vi "layout.vi"(0 "reference":refnum<class "CallNode.lvclass">, 1 "graph":refnum<class "Graph.lvclass">, 2 "graphics":refnum<class "Graphics.lvclass">, 3 "grid":refnum<class "Grid.lvclass">, 5 "error in (no error)":errorcluster) -> (14 "reference out":refnum<class "CallNode.lvclass">, 19 "error out":errorcluster)   [LabVIEW 2016, in "CallNode.lvclass"]
doc: "public void layout(Graph g, Graphics2D g2, Grid grid)"
uses:
  <resource>/Framework/Providers/Open_GDS/UML/CallNode_class/CallNode.lvclass
  C:/Program Files (x86)/National Instruments/LabVIEW 2016/resource/Framework/Providers/Open_GDS/UML/RectangularNode_class/RectangularNode.lvclass
  C:/Program Files (x86)/National Instruments/LabVIEW 2016/resource/Framework/Providers/Open_GDS/UML/AbstractNode_class/AbstractNode.lvclass
  <resource>/Framework/Providers/Open_GDS/UML/Graph_class/Graph.lvclass
  <resource>/Framework/Providers/Open_GDS/UML/Graphics_class/Graphics.lvclass
  <resource>/Framework/Providers/Open_GDS/UML/Grid_class/Grid.lvclass
  <resource>/Framework/Providers/Open_GDS/UML/ImplicitParameterNode_class/ImplicitParameterNode.lvclass
  <resource>/Framework/Providers/Open_GDS/UML/AbstractNode_class/AbstractNode.lvclass
  <resource>/Framework/Providers/Open_GDS/UML/RectangularNode_class/RectangularNode.lvclass
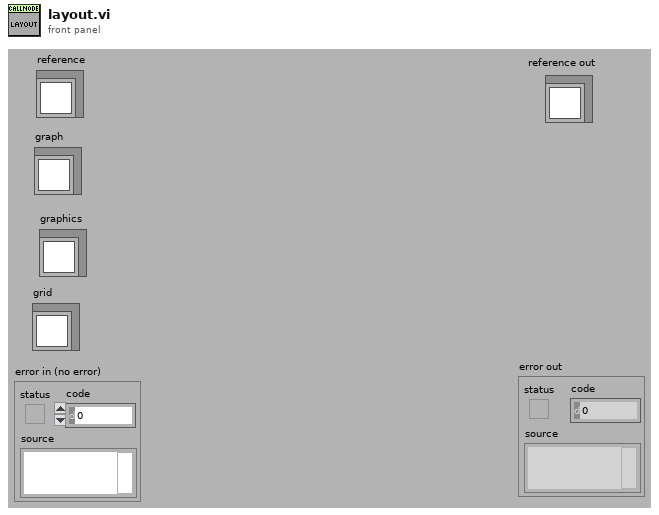
[diagram p1: front panel]
types:
  T1 = typedef "CallNode.lvclass/ObjectAttributes.ctl" = cluster{"objectCallNodeRef":refnum<class "AbstractNode.lvclass">, "signaled":bool, "openBottom":bool, "DEFAULT_WIDTH":i32, "DEFAULT_HEIGHT":i32, "CALL_YGAP":i32}
  T2 = typedef "RectangularNode.lvclass/ObjectAttributes.ctl" = cluster{"bounds":T3}
  T3 = typedef "Rectangle Rectangle2D.ctl" = cluster{"x":dbl, "y":dbl, "width":dbl, "height":dbl}
  T4 = typedef "AbstractNode.lvclass/ObjectAttributes.ctl" = cluster{"parent":refnum<class "AbstractNode.lvclass">, "children":refnum<class "AbstractNode.lvclass">[], "Hidden":bool}
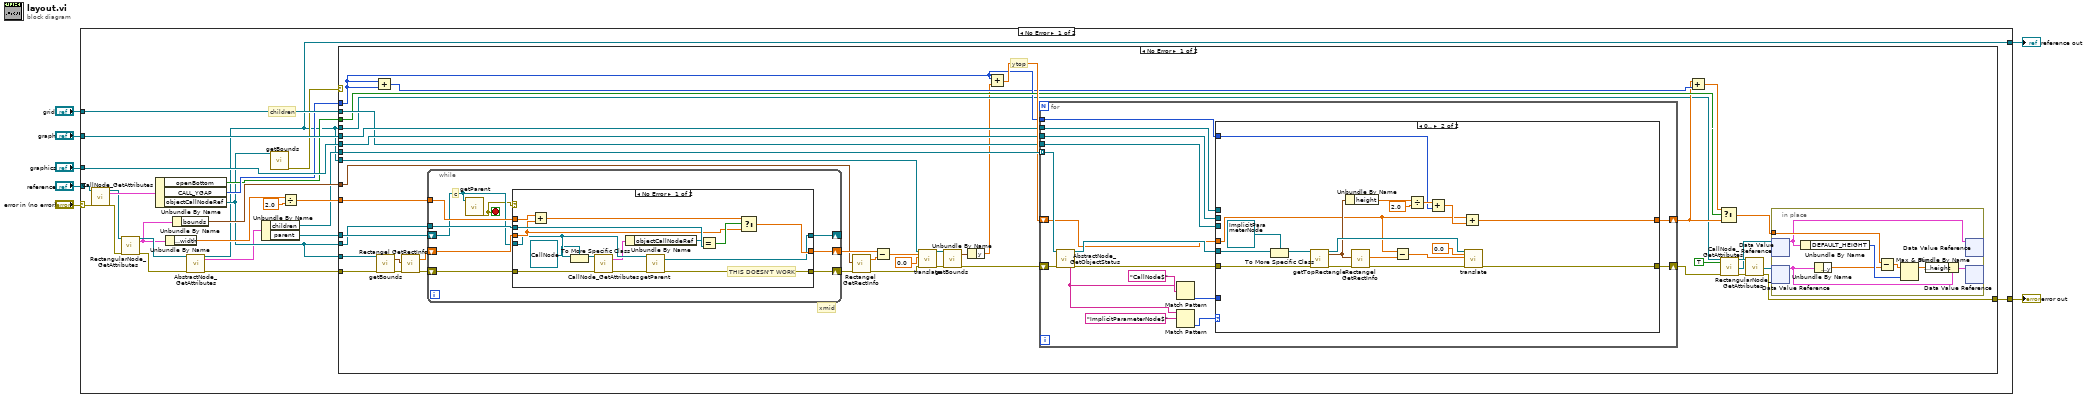
[diagram p0: block diagram]
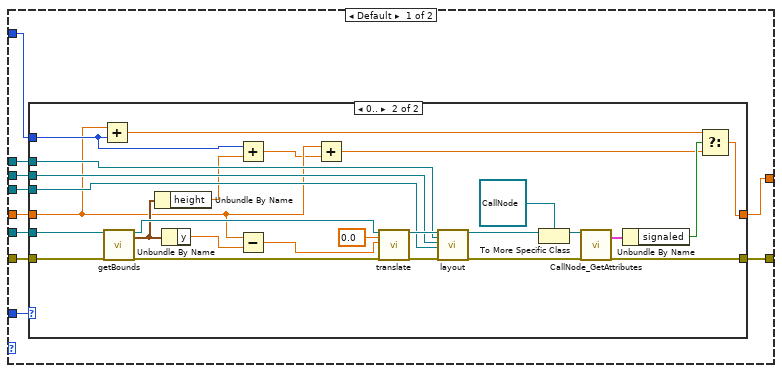
[diagram p2: hidden frame]
diagram:
  n1 = case shown="No Error" "error in (no error)" {
    selector: "error in (no error)" -> [w30 w184]
    tunnel: "reference" -> [w32 w185]
    tunnel: [w31 w184] -> w6
    tunnel: [w10 w185] -> w5
    tunnel: "graph" -> [w29 _]
    tunnel: "graphics" -> [w28 _]
    tunnel: "grid" -> [w27 _]
    frame No Error {
      # "children"
      n2 = call <resource>:"CallNode_GetAttributes.vi"("reference in"=w32, "error in (no error)"=w30) -> ("reference out"=w15:refnum<class "CallNode.lvclass">, "Data"=w16:T1, "error out"=w14:errorcluster)  [unwired: 1 in, 14 out]
      n3 = call <resource>:"RectangularNode_GetAttributes.vi"("reference in"=w15, "error in (no error)"=w14) -> ("reference out"=w13:refnum<class "CallNode.lvclass">, "Data"=w9:T2, "error out"=w12:errorcluster)  [unwired: 14 in, 1 out]
      n4 = Unbundle By Name(w16) -> ("openBottom"=w19:bool, "CALL_YGAP"=w21:i32, "objectCallNodeRef"=w17:refnum<class "AbstractNode.lvclass">)
      n5 = Unbundle By Name(w9) -> ("bounds.width"=w25:dbl)
      n6 = Unbundle By Name(w9) -> ("bounds"=w22:T3)
      n7 = call <resource>:"AbstractNode_GetAttributes.vi"("reference in"=w13, "error in (no error)"=w12) -> ("reference out"=w10:refnum<class "CallNode.lvclass">, "Data"=w8:T4, "error out"=w11:errorcluster)  [unwired: 14 in, 1 out]
      n8 = Unbundle By Name(w8) -> ("children"=w20:refnum<class "AbstractNode.lvclass">[], "parent"=w26:refnum<class "AbstractNode.lvclass">)
      n9 = call-dynamic "getBounds.vi"("reference"=w17) -> ("error out"=w18:errorcluster)  [unwired: 16 in, 2 out]
      n10 = Divide(x=w25, y=2.0) -> (x/y=w23:dbl)
      n11 = case shown="No Error" w18 {
        tunnel: w11 -> [w72 w183]
        tunnel: [w46 w183] -> w31
        tunnel: w17 -> [w73 _]
        tunnel: w26 -> [w69 _]
        tunnel: w17 -> [w67 _]
        tunnel: w23 -> [w65 _]
        tunnel: w10 -> [w64 _]
        tunnel: w22 -> [w58 _]
        tunnel: w21 -> [w51 _]
        tunnel: w20 -> [w57 _]
        tunnel: w29 -> [w55 _]
        tunnel: w28 -> [w54 _]
        tunnel: w27 -> [w53 _]
        tunnel: w19 -> [w52 _]
        tunnel: w10 -> [w47 _]
        frame No Error {
          # "ytop"
          # "xmid"
          n12 = Add(x=w51, y=w51) -> (x+y=w50:i32)
          n13 = call-dynamic "getBounds.vi"("reference"=w73, "error in (no error)"=w72) -> ("bounds"=w71:T3, "error out"=w70:errorcluster)  [unwired: 15 in, 1 out]
          n14 = call <resource>:"Rectangel GetRectInfo.vi"("bounds"=w71, "error in (no error)"=w70) -> ("centerX"=w66:dbl, "error out"=w68:errorcluster)  [unwired: 16 out]
          n15 = while {
            shift-right: [w159] -> _
            shift-left: w69 -> [w157]
            shift-right: [w158] -> w44
            shift-left: w68 -> [w160]
            tunnel: w67 -> [w164]
            shift-right: [w162] -> w62
            shift-left: w66 -> [w163]
            tunnel: w65 -> [w161]
            stop <- w156 stop-if-true
            # "c"
            n16 = call-dynamic "getParent.vi"("reference"=w157) -> ("error out"=w156:errorcluster)  [unwired: 14 in, 4 out]
            n17 = case shown="No Error" w156 {
              tunnel: w164 -> [w179 _]
              tunnel: w163 -> [w175 w182]
              tunnel: [w176 w182] -> w162
              tunnel: w161 -> [w174 _]
              tunnel: w160 -> [w172 w181]
              tunnel: w157 -> [w168 w180]
              tunnel: [w171 w180] -> w159
              tunnel: [w169 w181] -> w158
              frame No Error {
                # "THIS DOESN'T WORK"
                n18 = Add(x=w174, y=w175) -> (x+y=w173:dbl)
                n19 = To More Specific Class(target class=refnum<class "CallNode.lvclass"> refnum ("reference in"), reference=w168) -> (specific class reference=w166:refnum<class "CallNode.lvclass">)  [unwired: 1 in, 1 out]
                n20 = call <resource>:"CallNode_GetAttributes.vi"("reference in"=w166, "error in (no error)"=w172) -> ("Data"=w165:T1, "error out"=w170:errorcluster)  [unwired: 1 in, 15 out]
                n21 = Unbundle By Name(w165) -> ("objectCallNodeRef"=w178:refnum<class "AbstractNode.lvclass">)
                n22 = call-dynamic "getParent.vi"("reference"=w168, "error in (no error)"=w170) -> ("parentNode"=w171:refnum<class "AbstractNode.lvclass">, "error out"=w169:errorcluster)  [unwired: 13 in, 3 out]
                n23 = Equal?(x=w178, y=w179) -> (x = y?=w177:bool)
                n24 = Select(t=w173, s=w177, f=w175) -> (s? t:f=w176:dbl)
              }
              frame Error {
              }
            }
          }
          n25 = call <resource>:"Rectangel GetRectInfo.vi"("bounds"=w58, "error in (no error)"=w44) -> ("centerX"=w61:dbl, "error out"=w63:errorcluster)  [unwired: 16 out]
          n26 = Subtract(x=w62, y=w61) -> (x-y=w60:dbl)
          n27 = call-dynamic "translate.vi"("reference"=w64, "dx"=w60, "dy"=0.0, "error in (no error)"=w63) -> ("reference out"=w43:refnum<class "CallNode.lvclass">, "error out"=w42:errorcluster)  [unwired: 14 in]
          n28 = call-dynamic "getBounds.vi"("reference"=w43, "error in (no error)"=w42) -> ("bounds"=w40:T3, "error out"=w41:errorcluster)  [unwired: 15 in, 1 out]
          n29 = Unbundle By Name(w40) -> ("y"=w39:dbl)
          n30 = Add(x=w51, y=w39) -> (x+y=w56:dbl)
          n31 = for {
            tunnel: w57 -> [w97] mode=indexing
            shift-right: [w86] -> w45
            shift-left: w41 -> [w96]
            shift-right: [w90] -> w49
            shift-left: w56 -> [w82]
            tunnel: w51 -> [w91]
            tunnel: w55 -> [w85]
            tunnel: w54 -> [w84]
            tunnel: w53 -> [w83]
            n32 = call <resource>:"AbstractNode_GetObjectStatus.vi"("reference in"=w97, "error in (no error)"=w96) -> ("Class name"=w88:string, "reference out"=w92:refnum<class "AbstractNode.lvclass">, "error out"=w93:errorcluster)  [unwired: 15 out]
            n33 = Match Pattern(string=w88, regular expression="CallNode$") -> (offset past match=w87:i32)  [unwired: 4 out]
            n34 = Match Pattern(string=w88, regular expression="ImplicitParameterNode$") -> (offset past match=w94:i32)  [unwired: 4 out]
            n35 = case shown="0.." w94 {
              tunnel: w93 -> [w105 w155]
              tunnel: w92 -> [w106 w139]
              tunnel: w82 -> [w104 w142]
              tunnel: w91 -> [w100 w144]
              tunnel: [w99 w141] -> w90
              tunnel: w87 -> [w107 _]
              tunnel: [w98 w140] -> w86
              tunnel: w85 -> [w103 _]
              tunnel: w84 -> [w102 _]
              tunnel: w83 -> [w101 _]
              frame Default {
                n36 = case shown="0.." w107 {
                  tunnel: w106 -> [_ w136]
                  tunnel: w105 -> [w109 w135]
                  tunnel: w104 -> [w108 w118]
                  tunnel: w103 -> [_ w127]
                  tunnel: w102 -> [_ w126]
                  tunnel: w101 -> [_ w125]
                  tunnel: w100 -> [_ w119]
                  tunnel: [w108 w114] -> w99
                  tunnel: [w109 w121] -> w98
                  frame Default {
                  }
                  frame 0.. {
                    n37 = Add(x=w118, y=w119) -> (x+y=w122:dbl)
                    n38 = call-dynamic "getBounds.vi"("reference"=w136, "error in (no error)"=w135) -> ("reference out"=w134:refnum<class "AbstractNode.lvclass">, "bounds"=w132:T3, "error out"=w133:errorcluster)  [unwired: 15 in]
                    n39 = Unbundle By Name(w132) -> ("height"=w120:dbl)
                    n40 = Unbundle By Name(w132) -> ("y"=w131:dbl)
                    n41 = Add(x=w119, y=w120) -> (x+y=w117:dbl)
                    n42 = Subtract(x=w118, y=w131) -> (x-y=w115:dbl)
                    n43 = Add(x=w118, y=w117) -> (x+y=w116:dbl)
                    n44 = call-dynamic "translate.vi"("reference"=w134, "dx"=0.0, "dy"=w115, "error in (no error)"=w133) -> ("reference out"=w128:refnum<class "AbstractNode.lvclass">, "error out"=w129:errorcluster)  [unwired: 14 in]
                    n45 = call-dynamic "layout.vi"("reference"=w128, "graph"=w127, "graphics"=w126, "grid"=w125, "error in (no error)"=w129) -> ("reference out"=w113:refnum<class "AbstractNode.lvclass">, "error out"=w124:errorcluster)  [unwired: 13 in]
                    n46 = To More Specific Class(target class=refnum<class "CallNode.lvclass"> refnum ("reference out"), reference=w113) -> (specific class reference=w112:refnum<class "CallNode.lvclass">)  [unwired: 1 in, 1 out]
                    n47 = call <resource>:"CallNode_GetAttributes.vi"("reference in"=w112, "error in (no error)"=w124) -> ("Data"=w110:T1, "error out"=w121:errorcluster)  [unwired: 1 in, 15 out]
                    n48 = Unbundle By Name(w110) -> ("signaled"=w123:bool)
                    n49 = Select(t=w122, s=w123, f=w116) -> (s? t:f=w114:dbl)
                  }
                }
              }
              frame 0.. {
                n50 = To More Specific Class(target class=refnum<class "ImplicitParameterNode.lvclass"> refnum ("reference"), reference=w139) -> (specific class reference=w137:refnum<class "ImplicitParameterNode.lvclass">)  [unwired: 1 in, 1 out]
                n51 = call-dynamic "getTopRectangle.vi"("reference"=w137, "error in (no error)"=w155) -> ("reference out"=w152:refnum<class "ImplicitParameterNode.lvclass">, "bounds"=w148:T3, "error out"=w154:errorcluster)  [unwired: 15 in]
                n52 = Unbundle By Name(w148) -> ("height"=w147:dbl)
                n53 = call <resource>:"Rectangel GetRectInfo.vi"("bounds"=w148, "error in (no error)"=w154) -> ("centerY"=w153:dbl, "error out"=w149:errorcluster)  [unwired: 16 out]
                n54 = Subtract(x=w142, y=w153) -> (x-y=w151:dbl)
                n55 = Divide(x=w147, y=2.0) -> (x/y=w145:dbl)
                n56 = Add(x=w145, y=w144) -> (x+y=w143:dbl)
                n57 = Add(x=w142, y=w143) -> (x+y=w141:dbl)
                n58 = call-dynamic "translate.vi"("reference"=w152, "dx"=0.0, "dy"=w151, "error in (no error)"=w149) -> ("error out"=w140:errorcluster)  [unwired: 14 in, 1 out]
              }
            }
          }
          n59 = Add(x=w49, y=w50) -> (x+y=w48:dbl)
          n60 = Select(t=w48, s=w52, f=w49) -> (s? t:f=w33:dbl)
          n61 = call <resource>:"CallNode_GetAttributes.vi"("reference in"=w47, "OnlyGetDvrReference(False)"=TRUE, "error in (no error)"=w45) -> ("reference out"=w37:refnum<class "CallNode.lvclass">, "DataRef"=w35:refnum<data-value>, "error out"=w36:errorcluster)  [unwired: 13 in, 1 out]
          n62 = call <resource>:"RectangularNode_GetAttributes.vi"("reference in"=w37, "error in (no error)"=w36) -> ("DataRef"=w34:refnum<data-value>, "error out"=w46:errorcluster)  [unwired: 14 in, 2 out]
          n63 = in-place {
            in-place-border: w33 -> [w75]
            n64 = in-place-dvr #1(w35) -> (w74:T1)  [unwired: 1 out]
            n65 = in-place-dvr #2(w34) -> (w78:T2)  [unwired: 1 out]
            n66 = Unbundle By Name(w74) -> ("DEFAULT_HEIGHT"=w81:i32)
            n67 = Unbundle By Name(w78) -> ("bounds.y"=w76:dbl)
            n68 = Subtract(x=w75, y=w76) -> (x-y=w80:dbl)
            n69 = Max & Min(x=w80, y=w81) -> (max(x,y)=w79:dbl)  [unwired: 1 out]
            n70 = Bundle By Name(cluster=w78, "bounds.height"=w79) -> (w77:T2)
            n71 = in-place-dvr #1(w74) -> ()  [unwired: 2 out]
            n72 = in-place-dvr #2(w77) -> ()  [unwired: 2 out]
          }
        }
        frame Error {
          # "return"
        }
      }
    }
    frame Error {
    }
  }
  "reference out" <- w5
  "error out" <- w6
